vi "Play Path.vi"(6 "Synchronication":enum16{"Start", "Wait"}(ring), 7 "Description":string, 8 "Command Info In":T1, 10 "Reset Gyro":bool=TRUE, 11 "Path":path) -> (0 "Command Info Out":T1)   [LabVIEW 2019]
doc: "This VI notifies the subsystem to the new setpoint."
uses:
  <vilib>/Rock Robotics/WPI/Framework/Command Status Info.ctl
  <vilib>/Rock Robotics/WPI/Framework/Completion Status.ctl
  <vilib>/Rock Robotics/WPI/Framework/Completion Notifier.ctl
  Implementation/Drive Setpoints.ctl
  Implementation/Drive Operations.ctl
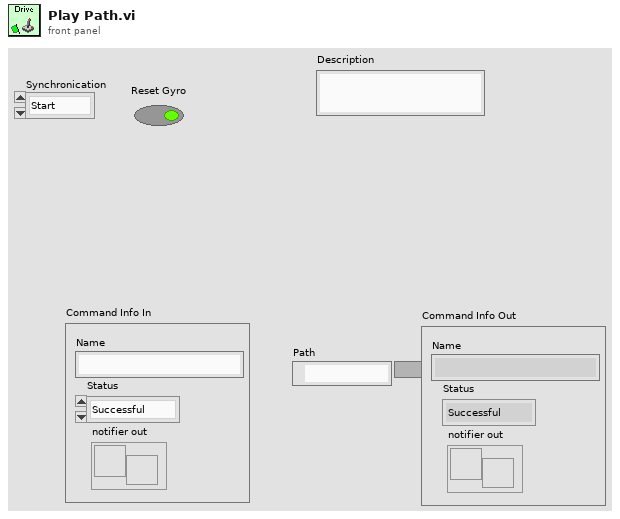
[diagram p1: front panel]
types:
  T1 = typedef "Command Status Info.ctl" = cluster{"Name":string, "Status":T2, "notifier out":T3}
  T2 = typedef "Completion Status.ctl" = enum16{"Successful", "Aborted", "Incomplete"}
  T3 = typedef "Completion Notifier.ctl" = refnum<notifier>
  T4 = typedef "Drive Operations.ctl" = enum16{"Reserve", "Read Current", "Immediate", "Drive for Time", "Drive for Distance", "Play Path"}
  T5 = cluster{"V":dbl[], "Theta":dbl[], "Sample Period":dbl}
  T6 = typedef "Drive Setpoints.ctl" = cluster{"Operation":T4, "Left Setpoint":dbl, "Right Setpoint":dbl, "Auto Path Data":cluster{"V":dbl[], "Theta":dbl[], "Sample Period":dbl}, "Reset Gyro?":bool, "Path Playback/Direction":cluster{"Robot Backwards":bool, "Reverse Path":bool}}
  T7 = cluster{"Robot Backwards":bool, "Reverse Path":bool}
  T8 = cluster{"Sample Period (s)":dbl, "Velocity Limit (fps)":dbl, "Acceleration Limit (fps^2)":dbl}
  T9 = cluster{"Segment Name":string, "Type":enum16{"Accel Straight", "Const Straight", "Blend", "Circle"}, "Traj Pos Points":cluster{"x":dbl, "y":dbl, "th":dbl}[], "Traj Vel Points":cluster{"V":dbl, "th":dbl}[], "Accel Index":i32, "Decel Index":i32}[]
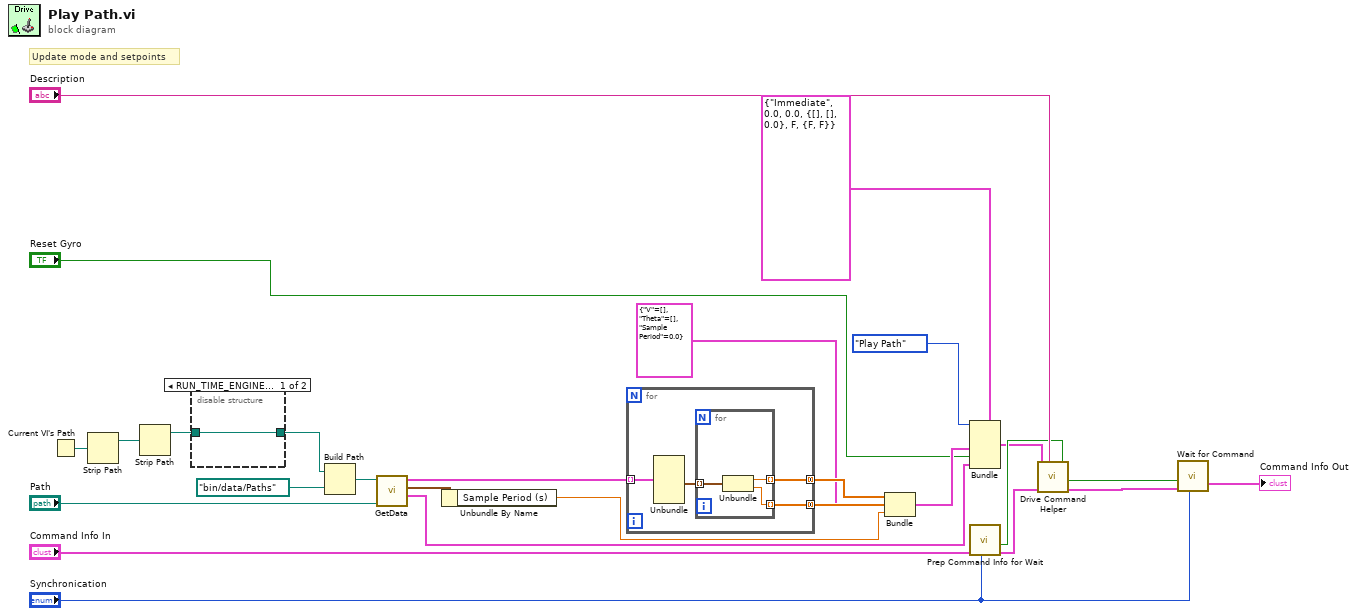
[diagram p0: block diagram]
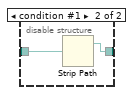
[diagram p2: hidden frame]
diagram:
  # "Update mode and setpoints"
  n1 = Current VI's Path() -> (path=w16:path)
  n2 = Strip Path(path=w16) -> (stripped path=w15:path)  [unwired: 1 out]
  n3 = Strip Path(path=w15) -> (stripped path=w12:path)  [unwired: 1 out]
  n4 = disable-structure shown="RUN_TIME_ENGINE==False" {
    disable-tunnel: [w27 w28] -> w13
    disable-tunnel: w12 -> [w27 w29]
    frame condition #0 (active) {
    }
    frame condition #1 {
      n5 = Strip Path(path=w29) -> (stripped path=w28:path)  [unwired: 1 out]
    }
  }
  n6 = Build Path(base path=w13, name or relative path=path "bin/data/Paths") -> (appended path=w17:path)
  n7 = call "GetData.vi"("file (use dialog) 2"="Path", "file (use dialog)"=w17) -> ("Path Playback/Direction"=w2:T7, "Trajectory Limits"=w4:T8, "Trajectory Data"=w18:T9)  [unwired: 3 in, 4 out]
  n8 = Unbundle By Name(w4) -> ("Sample Period (s)"=w3:dbl)
  n9 = for {
    tunnel: [w33] -> w11 mode=concatenating
    tunnel: [w32] -> w10 mode=concatenating
    tunnel: w18 -> [w30] mode=indexing
    n10 = Unbundle(w30) -> ("Traj Vel Points"=w31:cluster{"V":dbl, "th":dbl}[])  [unwired: 5 out]
    n11 = for {
      tunnel: w31 -> [w34] mode=indexing
      tunnel: [w36] -> w33 mode=indexing
      tunnel: [w35] -> w32 mode=indexing
      n12 = Unbundle(w34) -> ("V"=w36:dbl, "th"=w35:dbl)
    }
  }
  n13 = Bundle(cluster=T5 {"V"=[], "Theta"=[], "Sample Period"=0.0} ("Auto Path Data"), "V"=w11, "Theta"=w10, "Sample Period"=w3) -> (w5:T5)
  n14 = Bundle(cluster=T6 {"Operation"=enum."Immediate", "Left Setpoint"=0.0, "Right Setpoint"=0.0, "Auto Path Data"={"V"=[], "Theta"=[], "Sample Period"=0.0}, "Reset Gyro?"=FALSE, "Path Playback/Direction"={"Robot Backwards"=FALSE, "Reverse Path"=FALSE}} ("SubSystem Data"), "Operation"=Drive_Operations."Play Path", "Auto Path Data"=w5, "Reset Gyro?"="Reset Gyro", "Path Playback/Direction"=w2) -> (w6:T6)  [unwired: 2 in]
  n15 = call <vilib>:"Prep Command Info for Wait.vi"("Synchronication"="Synchronication", "Command Info"="Command Info In") -> ("Command Info"=w24:T1, "Allocated"=w20:bool)  [unwired: 8 in]
  n16 = call "Drive Command Helper.vi"("Description"="Description", "Command Info In"=w24, "SubSystem Data"=w6) -> ("Command Info Out"=w23:T1)  [unwired: 6 in, 2 out]
  n17 = call <vilib>:"Wait for Command.vi"("Synchronication"="Synchronication", "Command Info in"=w23, "Allocated"=w20) -> ("Command Info out"=→"Command Info Out":T1)  [unwired: 8 in]
